vi "Vision Begin.vi"() -> (0 "Match Geometric Pattern 2 Setup Data":string, 1 "Gray Image":T1, 2 "Tempalte":T1, 3 "Mask":T1)   [LabVIEW 2014]
uses:
  <vilib>/vision/Image Controls.llb/IMAQ Image.ctl
  <vilib>/vision/Pattern Matching.llb/IMAQ Match Range Setting.ctl
  <vilib>/vision/Pattern Matching.llb/IMAQ Curve Parameters.ctl
  <vilib>/vision/NI_Vision_Development_Module.lvlib
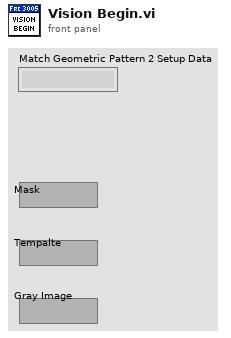
[diagram p1: front panel]
types:
  T1 = typedef "IMAQ Image.ctl" = refnum<image>
  T2 = cluster{"Rotation":bool, "Scale":bool, "Occlusion":bool, "Reserved":bool, "Reserved":bool, "Reserved":bool}
  T3 = typedef "IMAQ Curve Parameters.ctl" = cluster{"Extraction Mode":u32, "Edge Threshold":i32, "Edge Filter Size":u32, "Min Length":i32, "Row Search Step Size":i32, "Col Search Step Size":i32, "Max Endpoint Gap":i32, "Closed":bool, "Subpixel":bool}
  T4 = typedef "IMAQ Match Range Setting.ctl" = cluster{"Match Constraints":u32, "Min":dbl, "Max":dbl}
  T5 = typedef "Image Type" = u32
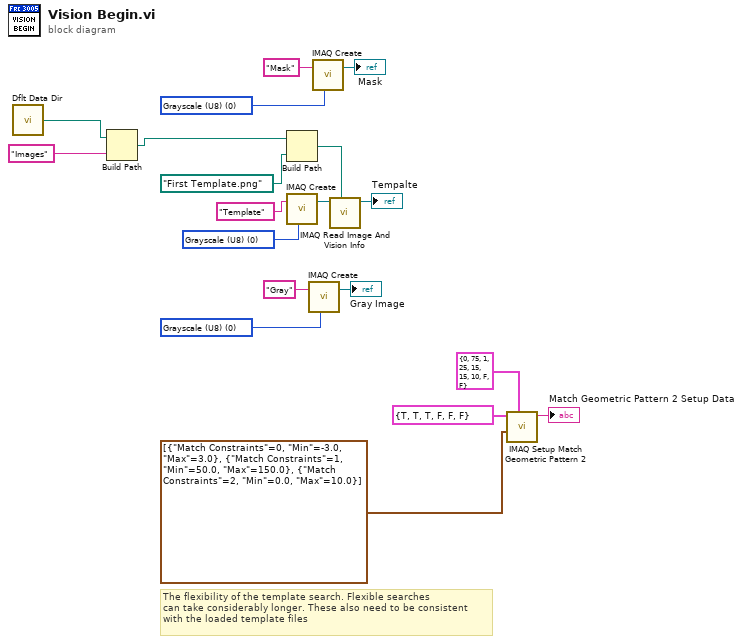
[diagram p0: block diagram]
diagram:
  w9 = T5 0 items=["Grayscale (U8)", "Grayscale (I16)", "Grayscale (SGL)", "Complex (CSG)", "RGB (U32)", "HSL (U32)", "RGB (U64)", "Grayscale (U16)"] ("Image Type")
  w7 = T5 0 items=["Grayscale (U8)", "Grayscale (I16)", "Grayscale (SGL)", "Complex (CSG)", "RGB (U32)", "HSL (U32)", "RGB (U64)", "Grayscale (U16)"] ("Image Type")
  w4 = T5 0 items=["Grayscale (U8)", "Grayscale (I16)", "Grayscale (SGL)", "Complex (CSG)", "RGB (U32)", "HSL (U32)", "RGB (U64)", "Grayscale (U16)"] ("Image Type")
  # "The flexibility of the template search. Flexible searches\ncan take considerably longer. These also need to be consistent\nwith the loaded template files"
  n1 = call <vilib>:"Dflt Data Dir.vi"() -> ("App:Default Data Directory"=w2:path)
  n2 = Build Path(base path=w2, name or relative path="Images") -> (appended path=w1:path)
  n3 = Build Path(base path=w1, name or relative path=path "First Template.png") -> (appended path=w19:path)
  n4 = call "IMAQ Create"("Image Name"="Template", "Image Type"=w9) -> ("New Image"=w17:T1)  [unwired: 2 in, 2 out]
  n5 = call "IMAQ Create"("Image Name"="Gray", "Image Type"=w7) -> ("New Image"=→"Gray Image":T1)  [unwired: 2 in, 2 out]
  n6 = call "IMAQ Create"("Image Name"="Mask", "Image Type"=w4) -> ("New Image"=→"Mask":T1)  [unwired: 2 in, 2 out]
  n7 = call "IMAQ Read Image And Vision Info"("File Path"=w19, "Image"=w17) -> ("Image Out"=→"Tempalte":T1)  [unwired: 2 in, 7 out]
  n8 = call "IMAQ Setup Match Geometric Pattern 2"("Curve Parameters"=T3 {"Extraction Mode"=0, "Edge Threshold"=75, "Edge Filter Size"=1, "Min Length"=25, "Row Search Step Size"=15, "Col Search Step Size"=15, "Max Endpoint Gap"=10, "Closed"=FALSE, "Subpixel"=FALSE}, "Range Settings"=T4[] [{"Match Constraints"=0, "Min"=-3.0, "Max"=3.0}, {"Match Constraints"=1, "Min"=50.0, "Max"=150.0}, {"Match Constraints"=2, "Min"=0.0, "Max"=10.0}], "Match Mode"=T2 {"Rotation"=TRUE, "Scale"=TRUE, "Occlusion"=TRUE, "Reserved"=FALSE, "Reserved"=FALSE, "Reserved"=FALSE}) -> ("Match Geometric Pattern 2 Setup Data"=→"Match Geometric Pattern 2 Setup Data":string)  [unwired: 7 in, 1 out]
